vi "test Read U16.vi"(8 "error in (no error)":errorcluster, 11 "TestCase in":refnum<class "Buffer Tests.lvclass">) -> (0 "error out":errorcluster, 3 "TestCase out":refnum<class "Buffer Tests.lvclass">)   [LabVIEW 2017, in "Buffer Tests.lvclass"]
uses:
  Buffer Tests.lvclass
  Classes/Buffer/Buffer.lvclass
  C:/Git/DSF/LabVIEW-Memory/Source/Classes/Pointer/Pointer.lvclass
  Classes/Buffer/Read Buffer 0D U16.vi
  <vilib>/addons/_JKI Toolkits/VI Tester/TestCase.llb/TestCase.lvclass
  LabVIEW-Memory/Source/Classes/Pointer/Pointer.lvclass
  C:/Program Files (x86)/National Instruments/LabVIEW 2017/vi.lib/addons/_JKI Toolkits/VI Tester/TestCase.llb/TestCase.lvclass
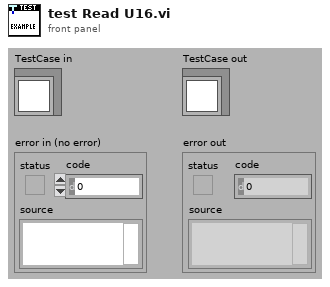
[diagram p1: front panel]
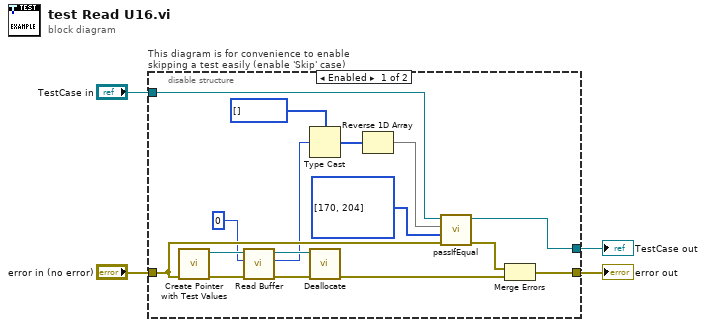
[diagram p0: block diagram]
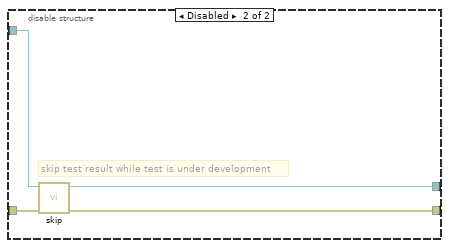
[diagram p2: hidden frame]
diagram:
  n1 = disable-structure "This diagram is for convenience to enable skipping a test easily (enable 'Skip' case)" shown="Enabled" {
    disable-tunnel: "TestCase in" -> [w13 w24]
    disable-tunnel: [w16 w22] -> w1
    disable-tunnel: [w11 w23] -> w2
    disable-tunnel: "error in (no error)" -> [w12 w21]
    frame Enabled {
      n2 = call "Create Pointer with Test Values.vi"("error in (no error)"=w12) -> ("error out"=w8:errorcluster, "Buffer out"=w6:refnum<class "Buffer.lvclass">)  [unwired: 9 in]
      n3 = call-poly "Read Buffer.vi"("error in (no error)"=w8, "dst value in"=u16 0, "Buffer in"=w6) -> ("error out"=w19:errorcluster, "dst value out"=w10:u16, "Buffer out"=w20:refnum<class "Buffer.lvclass">)  [unwired: 5 in, 1 out]
      n4 = Type Cast(type=u8[] [] ("buffer in"), x=w10) -> (*(type *) &x=w18:u8[])
      n5 = call "Deallocate.vi"("error in (no error)"=w19, "Pointer in"=w20) -> ("error out"=w7:errorcluster)  [unwired: 8 in, 1 out]
      n6 = Reverse 1D Array(array=w18) -> (reversed array=w14:u8[])
      n7 = call-dynamic "passIfEqual.vi"("error in (no error)"=w12, "y"=u8[] [170, 204] ("subarray 3"), "x"=w14, "TestCase in"=w13) -> ("error out"=w15:errorcluster, "TestCase out"=w16:refnum<class "Buffer Tests.lvclass">)  [unwired: 6 in]
      n8 = Merge Errors(w15, w7) -> (w11:errorcluster)
    }
    frame Disabled {
      # "skip test result while test is under development"
      n9 = call <vilib>:"skip.vi"("error in (no error)"=w21, "TestCase in"=w24) -> ("error out"=w23:errorcluster, "TestCase out"=w22:refnum<class "Buffer Tests.lvclass">)  [unwired: 8 in]
    }
  }
  "error out" <- w2
  "TestCase out" <- w1
